vi "ex_load event stack.vi"(7 "Number of Measurements":i32=6, 9 "Selected Measurements":u32) -> (1 "Array":i32[](array[numeric]))   [LabVIEW 2020]
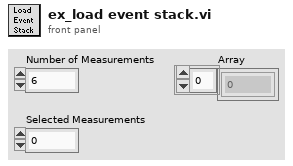
[diagram p1: front panel]
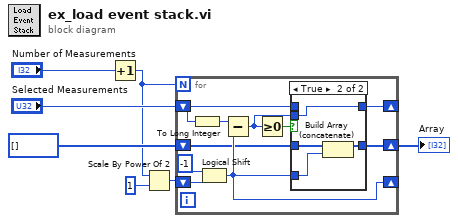
[diagram p0: block diagram]
diagram:
  n1 = Increment(x="Number of Measurements") -> (x+1=w1:i32)
  n2 = Scale By Power Of 2(n=w1, x=1) -> (x*2^n=w3:i32)
  n3 = for {
    N: w1 -> [_]
    shift-right: [w10] -> _
    shift-left: w3 -> [w15]
    shift-right: [w12] -> _
    shift-left: "Selected Measurements" -> [w13]
    shift-right: [w9] -> w7
    shift-left: i32[] [] -> [w8]
    n4 = To Long Integer(number=w13) -> (32bit integer=w16:i32)
    n5 = Logical Shift(y=-1, x=w15) -> (x << y=w10:i32)
    n6 = Subtract(x=w16, y=w10) -> (x-y=w11:i32)
    n7 = Greater Or Equal To 0?(x=w11) -> (x >= 0?=w14:bool)
    n8 = case shown="True" w14 {
      tunnel: w13 -> [w19 _]
      tunnel: [w19 w23] -> w12
      tunnel: w11 -> [_ w23]
      tunnel: w8 -> [w18 w22]
      tunnel: [w18 w20] -> w9
      tunnel: w10 -> [_ w21]
      frame False {
      }
      frame True {
        n9 = Build Array (concatenate)(w22, w21) -> (w20:i32[])
      }
    }
  }
  "Array" <- w7
